vi "Create Tag Reader.vi"(8 "error in (no error)":errorcluster, 11 "Enclave in":refnum<class "Enclave.lvclass">) -> (0 "error out":errorcluster, 2 "Tag Reader":refnum<class "Tag.lvclass">, 3 "Enclave out":refnum<class "Enclave.lvclass">)   [LabVIEW 2022 SP3, in "Enclave.lvlib" / "Enclave.lvclass"]
uses:
  Enclave.lvclass
  Tag/Tag.lvclass
  Enclave.lvclass/Enclave.ctl
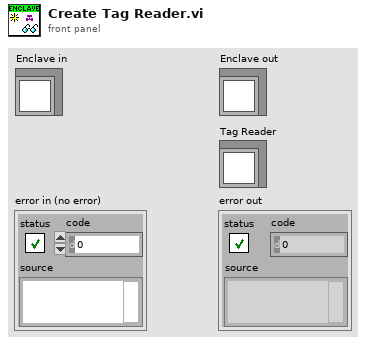
[diagram p1: front panel]
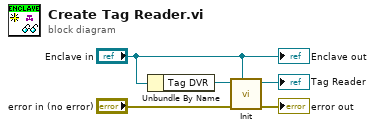
[diagram p0: block diagram]
diagram:
  n1 = Unbundle By Name("Enclave in") -> ("Tag DVR"=w3:refnum<data-value>)
  n2 = call "Init.vi"("Enclave"="Enclave in", "error in (no error)"="error in (no error)", "Tag DVR"=w3) -> ("error out"=→"error out":errorcluster, "Tag out"=→"Tag Reader":refnum<class "Tag.lvclass">)  [unwired: 7 in]
  "Enclave out" <- "Enclave in"
